vi "Global Data.vi"() -> ()   [LabVIEW 2014]
uses:
  SensorData.ctl
  navXPacket.ctl
  EncoderPacket.ctl
  PotentiometerPacket.ctl
  distanceSensorPacket.ctl
  switchPacket.ctl
  SensorType.ctl
  SensorStatus.ctl
  <vilib>/Rock Robotics/WPI/SerialPort/WPI_SerialPortRef.ctl
panel:
  in  "Packet Log":string[](array[string])
  out "SerialPortRef":T1
  in  "Array":T2[](array[typedef])
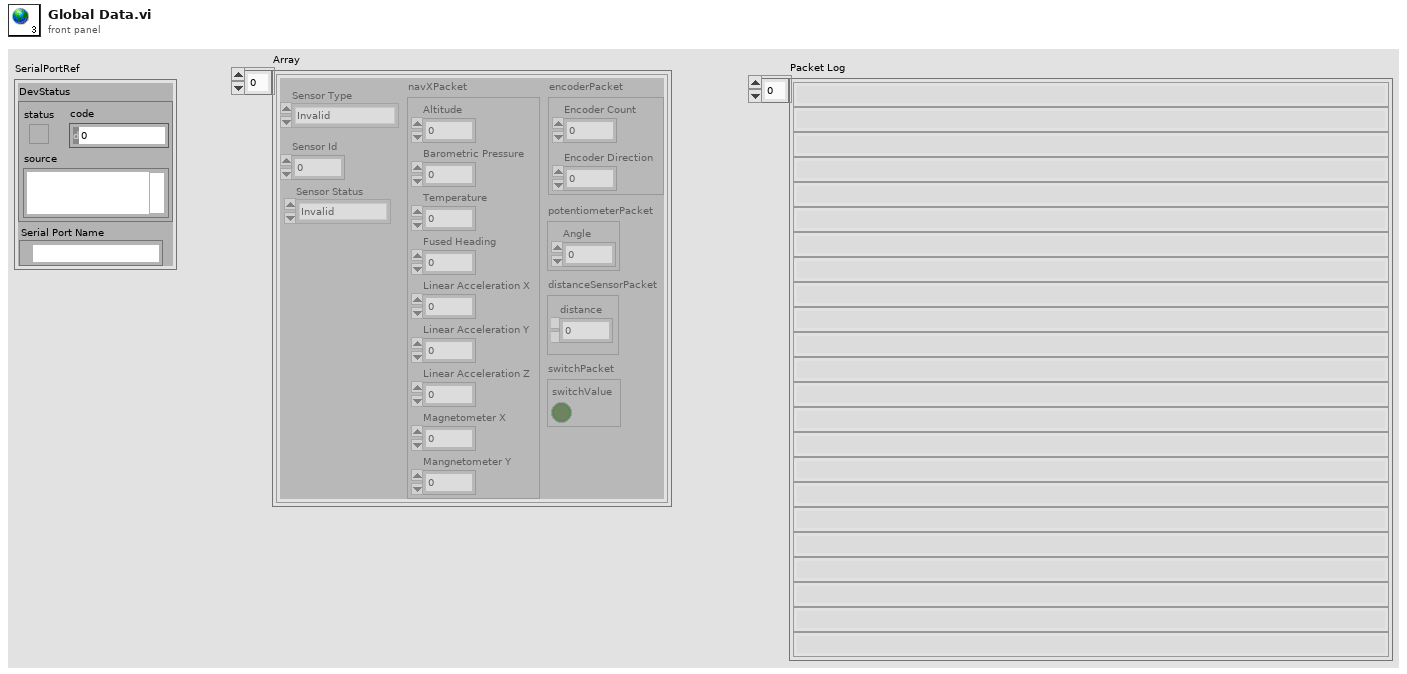
[diagram p1: front panel]
types:
  T1 = typedef "WPI_SerialPortRef.ctl" = cluster{"DevStatus":errorcluster, "Serial Port Name":refnum<visa-resource-name>}
  T2 = typedef "SensorData.ctl" = cluster{"Sensor Id":dbl, "navXPacket":T3, "encoderPacket":T4, "potentiometerPacket":T5, "distanceSensorPacket":T6, "switchPacket":T7, "Sensor Type":T8, "Sensor Status":T9}
  T3 = typedef "navXPacket.ctl" = cluster{"Altitude":dbl, "Barometric Pressure":dbl, "Fused Heading":dbl, "Linear Acceleration Y":dbl, "Linear Acceleration X":dbl, "Temperature":dbl, "Mangnetometer Y":dbl, "Magnetometer X":dbl, "Linear Acceleration Z":dbl}
  T4 = typedef "EncoderPacket.ctl" = cluster{"Encoder Count":dbl, "Encoder Direction":dbl}
  T5 = typedef "PotentiometerPacket.ctl" = cluster{"Angle":dbl}
  T6 = typedef "distanceSensorPacket.ctl" = cluster{"distance":dbl}
  T7 = typedef "switchPacket.ctl" = cluster{"switchValue":bool}
  T8 = typedef "SensorType.ctl" = enum16{"Invalid", "NavX", "Encoder", "Potentiometer", "Distance Sensor", "Switch"}
  T9 = typedef "SensorStatus.ctl" = enum16{"Invalid", "Operational", "Error occurred"}
diagram:
